vi "Manage collision.vi"(11 "Ball-Edge in":refnum<class "Ball-Edge.lvclass">) -> (1 "Remove GB Components out":refnum<class "Game Board Component.lvclass">[](array[class]), 2 "GB Components out":refnum<class "Game Board Component.lvclass">[](array[class]))   [LabVIEW 2021, in "Ball-Edge.lvclass"]
doc: "MIT Licence\nCopyright (c) 2024 David Grollier"
uses:
  Ball-Edge.lvclass
  C:/Users/David/Documents/GameSoccerSpace/Source/Collision/Collision.lvclass
  Game Componants/Game Board Component/Game Board Component.lvclass
  Collision.lvclass/Collision.ctl
  Ball-Edge.lvclass/Ball-Edge.ctl
  Game Componants/Game Board Component/Movable/Movable.lvclass/Movable.ctl
  Game Componants/Game Componants.lvclass/Game Componants.ctl
  Game Componants/Game Board Component/Movable/Movable.lvclass
  C:/Users/David/Documents/GameSoccerSpace/Source/Game Componants/Game Componants.lvclass
  C:/Users/David/Documents/GameSoccerSpace/Source/Game Componants/Game Board Component/Game Board Component.lvclass
  Game Componants/Game Board/Game Board.lvclass
  Collision.lvclass
  Game Componants/Game Componants.lvclass
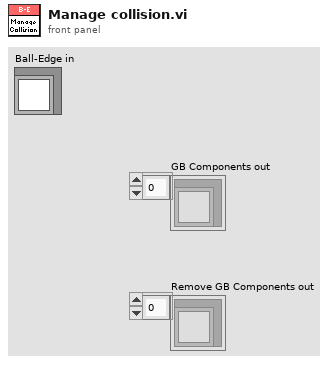
[diagram p1: front panel]
types:
  T1 = typedef "Ball-Edge.lvclass/Collision type.ctl" = enum16{"Horizontal", "Vertical", "Corner"}
  T2 = typedef "Velocity.ctl" = cluster{"Vx":dbl, "Vy":dbl}
  T3 = typedef "Coordinates.ctl" = cluster{"x":dbl, "y":dbl}
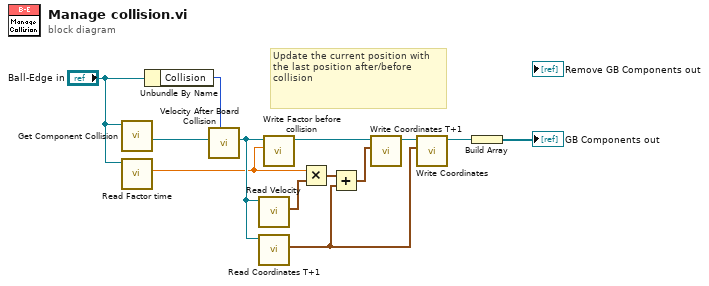
[diagram p0: block diagram]
diagram:
  # "Update the current position with the last position after/before collision"
  n1 = call "Get Component Collision.vi"("Collision in"="Ball-Edge in") -> ("Movable out"=w11:refnum<class "Movable.lvclass">)  [unwired: 9 in, 1 out]
  n2 = call "Read Factor time.vi"("Collision in"="Ball-Edge in") -> ("Factor time"=w1:dbl)  [unwired: 10 in]
  n3 = Unbundle By Name("Ball-Edge in") -> ("Collision"=w12:T1)
  n4 = call "Velocity After Board Collision.vi"("Collision in"=w12, "Movable in"=w11) -> ("Movable out"=w3:refnum<class "Movable.lvclass">)  [unwired: 9 in]
  n5 = call-dynamic "Read Velocity.vi"("Movable in"=w3) -> ("Velocity"=w7:T2)  [unwired: 10 in]
  n6 = call "Read Coordinates T+1.vi"("Movable in"=w3) -> ("Coordinates"=w8:T3)  [unwired: 10 in]
  n7 = call "Write Factor before collision.vi"("Factor before collision"=w1, "Movable in"=w3) -> ("Movable out"=w2:refnum<class "Movable.lvclass">)  [unwired: 9 in]
  n8 = Multiply(x=w1, y=w7) -> (x*y=w6:T2)
  n9 = Add(x=w6, y=w8) -> (x+y=w10:T2)
  n10 = call "Write Coordinates T+1.vi"("Coordinates"=w10, "Movable in"=w2) -> ("Movable out"=w9:refnum<class "Movable.lvclass">)  [unwired: 9 in]
  n11 = call "Write Coordinates.vi"("Coordinates"=w8, "Game Componants in"=w9) -> ("Game Componants out"=w5:refnum<class "Movable.lvclass">)  [unwired: 9 in]
  n12 = Build Array(w5) -> (→"GB Components out":refnum<class "Movable.lvclass">[])
